vi "DSF.Engine.Plugin.Set Transceiver Count.vi"(10 "transceiver count":i32, 11 "Plugin in":refnum<class "DSF.Engine.Plugin.lvclass">) -> (3 "Plugin out":refnum<class "DSF.Engine.Plugin.lvclass">)   [LabVIEW 2017, in "Data Sharing Framework Engine.lvlib" / "DSF.Engine.Plugin.lvclass"]
uses:
  DSF.Engine.Plugin.lvclass
  DSF.Engine.Plugin.lvclass/DSF.Engine.Plugin.ctl
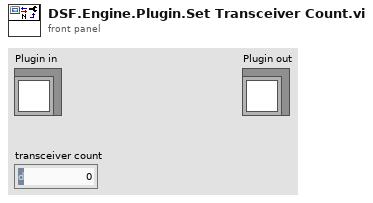
[diagram p1: front panel]
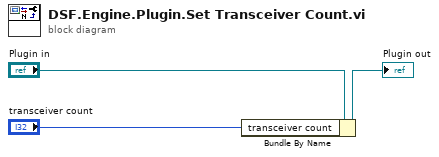
[diagram p0: block diagram]
diagram:
  n1 = Bundle By Name(cluster="Plugin in", "transceiver count"="transceiver count") -> (→"Plugin out":refnum<class "DSF.Engine.Plugin.lvclass">)
